vi "Move at Velocity.vi"(6 "Units (0: device speed units)":u16(ring) items=["device speed units", "microns per second", "millimeters per second", "inches per second", "degrees per second"], 7 "Velocity":dbl, 8 "error in (no error)":errorcluster, 9 "Device and Axis":string, 10 "Microstep Size (0)":dbl, 11 "VISA resource name":refnum<visa-resource-name>) -> (0 "error out":errorcluster, 3 "VISA resource name out":refnum<visa-resource-name>)   [LabVIEW 2015, in "Zaber A Series.lvlib"]
doc: "Moves a device at a specified velocity. If you select an input unit other than device speed units, you must also set the microstep size input to the physical size of your device's microstep in micrometers or degrees - consult your device's manual for this value.\n\nNo responses are returned with this VI, but if you would like to wait until the movement is completed to continue, you can combine this VI with the Poll Until Idle VI. \n\nMovement stops when the stage reaches the end of its travel or a stop command is received.\n\nThis VI requires that the Initialize VI has been called with the same serial port. \n\nNote: See the Device Lookup control for the microstep size of your model, or check on the product specifications page for the product on www.zaber.com."
uses:
  Zaber A Series.lvlib
  Private/Basic Commands.ctl
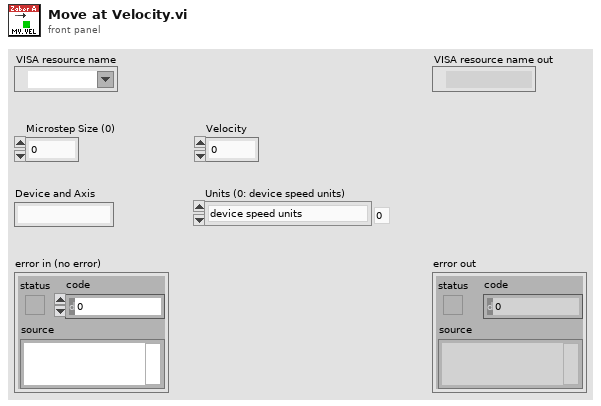
[diagram p1: front panel]
types:
  T1 = typedef "Zaber A Series.lvlib/Basic Commands.ctl" = string
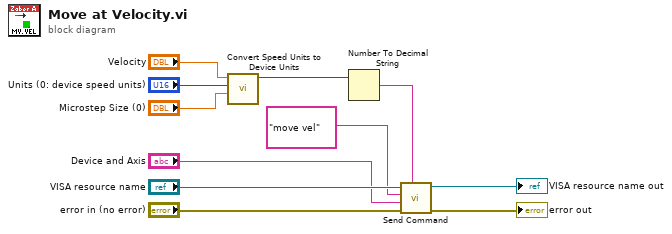
[diagram p0: block diagram]
diagram:
  n1 = call "Convert Speed Units to Device Units.vi"("Microstep Size (0)"="Microstep Size (0)", "Units (0: device speed units)"="Units (0: device speed units)", "Speed (0)"="Velocity") -> ("Device Speed (32-bit)"=w6:i32)  [unwired: 6 in, 2 out]
  n2 = Number To Decimal String(number=w6) -> (decimal integer string=w7:string)  [unwired: 1 in]
  n3 = call "Send Command.vi"("Data"=w7, "error in (no error)"="error in (no error)", "Device and Axis"="Device and Axis", "Command"=T1 "move vel" ("Basic Command List"), "VISA resource name"="VISA resource name") -> ("error out"=→"error out":errorcluster, "VISA resource name out"=→"VISA resource name out":refnum<visa-resource-name>)  [unwired: 1 in, 4 out]
